vi "NI_low_level_daq_analog_waveform_generator.vi"() -> ()   [LabVIEW 2025]
uses:
  <vilib>/DAQmx/write.llb/DAQmx Write (Analog 2D DBL NChan NSamp).vi
  <vilib>/DAQmx/create/channels.llb/DAQmx Create Channel (AO-Voltage-Basic).vi
  <vilib>/DAQmx/configure/timing.llb/DAQmx Timing (Sample Clock).vi
  <vilib>/DAQmx/miscellaneous.llb/DAQmx Fill In Error Info.vi
  <vilib>/measure/NI_MABase.lvlib
panel:
  in  "Number of Points":dbl=1000.0 format="%#_13g"
  in  "Sampling frequency":dbl=5000.0 format="%#_13g"
  in  "Together ON/OFF":bool
  out "Boolean":bool
  out "Boolean":bool
  in  "Output to DAQ":bool
  out "DAQ Output Voltage":waveform(dbl)[](graph)
  in  "Voltage Amplitude":i32=1 min=0 max=10 step=1
  in  "Frequency (Hz)":i32=10
  in  "Phase (degrees)":i32
  in  "Waveform":string(combo)="sine"
  in  "Phase (degrees)":i32
  in  "Waveform":string(combo)="sine"
  in  "Frequency (Hz)":i32=10
  in  "Voltage Amplitude":i32=1 min=0 max=10 step=1
  in  "stop":bool
  # "Waveform Generator (open-loop)"
  # "X-AXIS"
  # "Y-AXIS"
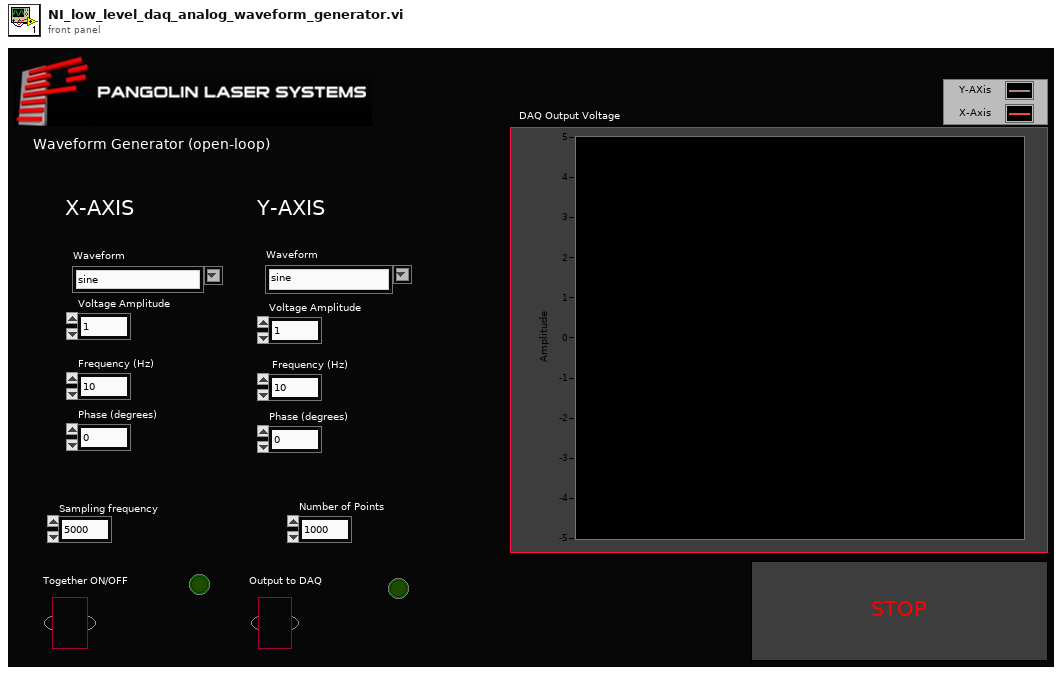
[diagram p1: front panel]
types:
  T1 = cluster{"Sampling frequency":dbl, "Number of Points":dbl}
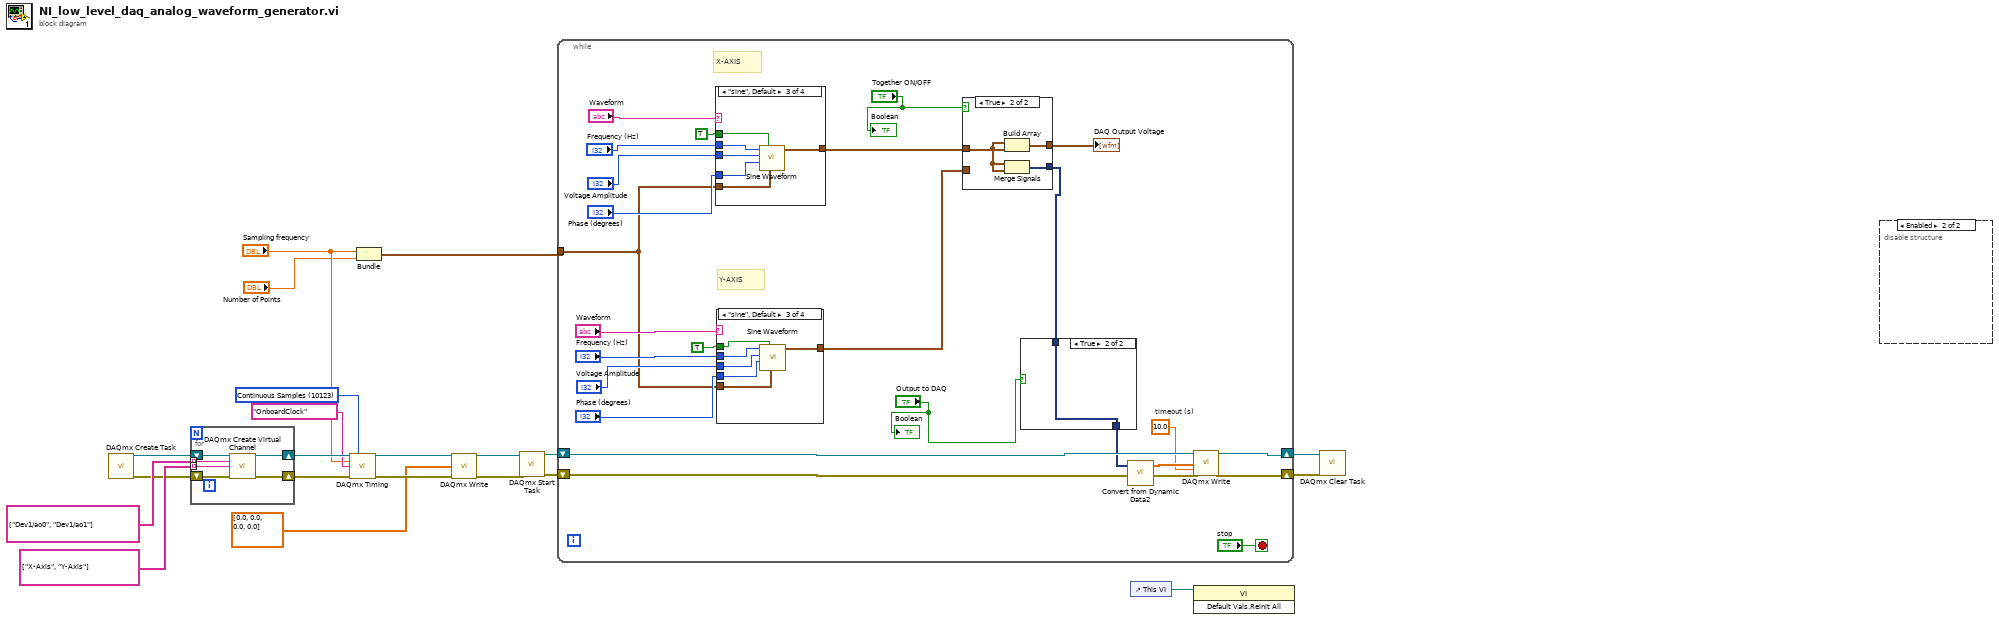
[diagram p0: block diagram]
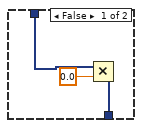
[diagram p2: hidden frame]
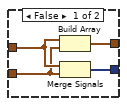
[diagram p3: hidden frame]
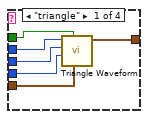
[diagram p4: hidden frame]
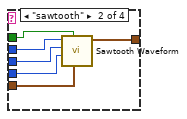
[diagram p5: hidden frame]
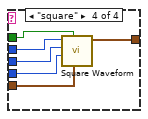
[diagram p6: hidden frame]
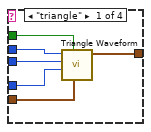
[diagram p7: hidden frame]
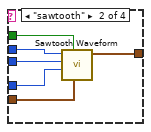
[diagram p8: hidden frame]
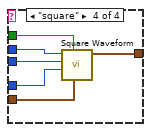
[diagram p9: hidden frame]
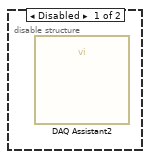
[diagram p10: hidden frame]
diagram:
  w14 = 10123 items=["Finite Samples"=10178, "Continuous Samples"=10123, "Hardware Timed Single Point"=12522] ("sample mode")
  n1 = call <vilib>:"DAQmx Create Task.vi"() -> ("task out"=w17:refnum<k21>, "error out"=w18:errorcluster)  [unwired: 14 in]
  n2 = for {
    tunnel: tag[] ["Dev1/ao0", "Dev1/ao1"] ("physical channels") -> [w27] mode=indexing
    tunnel: string[] ["X-Axis", "Y-Axis"] ("name to assign") -> [w26] mode=indexing
    shift-right: [w22] -> w15
    shift-left: w18 -> [w25]
    shift-right: [w23] -> w16
    shift-left: w17 -> [w24]
    n3 = call-poly <vilib>:"DAQmx Create Virtual Channel.vi"("task in"=w24, "physical channels"=w27, "name to assign"=w26, "error in"=w25) -> ("task out"=w23:refnum<k21>, "error out"=w22:errorcluster)  [unwired: 10 in]
  }
  n4 = call-poly <vilib>:"DAQmx Timing.vi"("task/channels in"=w16, "sample mode"=w14, "rate"="Sampling frequency", "source"=tag "OnboardClock", "error in"=w15) -> ("task out"=w11:refnum<k21>, "error out"=w10:errorcluster)  [unwired: 9 in]
  n5 = Bundle("Sampling frequency"="Sampling frequency", "Number of Points"="Number of Points") -> (w1:T1)  [unwired: 1 in]
  n6 = call-poly <vilib>:"DAQmx Write.vi"("task/channels in"=w11, "data"=dbl[][] [[0.0, 0.0], [0.0, 0.0]], "error in"=w10) -> ("task out"=w13:refnum<k21>, "error out"=w12:errorcluster)  [unwired: 10 in, 1 out]
  n7 = call <vilib>:"DAQmx Start Task.vi"("task/channels in"=w13, "error in"=w12) -> ("task out"=w8:refnum<k21>, "error out"=w6:errorcluster)  [unwired: 12 in]
  n8 = while {
    tunnel: w1 -> [w40]
    shift-right: [w50] -> w5
    shift-left: w8 -> [w52]
    shift-right: [w49] -> w4
    shift-left: w6 -> [w51]
    stop <- "stop" stop-if-true
    w30 = 10.0  # timeout (s)
    # "Y-AXIS"
    # "X-AXIS"
    n9 = case shown="\"sine\", Default" "Waveform" {
      tunnel: "Voltage Amplitude" -> [w92 w98 w104 w111]
      tunnel: "Frequency (Hz)" -> [w93 w99 w105 w110]
      tunnel: w40 -> [w89 w95 w102 w109]
      tunnel: [w90 w94 w101 w108] -> w38
      tunnel: "Phase (degrees)" -> [w91 w97 w103 w107]
      tunnel: TRUE ("reset signal") -> [w88 w96 w100 w106]
      frame "triangle" {
        n10 = call <vilib>:"Triangle Waveform.vi"("sampling info"=w89, "reset signal"=w88, "phase"=w91, "amplitude"=w92, "frequency"=w93) -> ("signal out"=w90:waveform(dbl))  [unwired: 5 in, 1 out]
      }
      frame "sawtooth" {
        n11 = call <vilib>:"Sawtooth Waveform.vi"("sampling info"=w95, "reset signal"=w96, "phase"=w97, "amplitude"=w98, "frequency"=w99) -> ("signal out"=w94:waveform(dbl))  [unwired: 5 in, 1 out]
      }
      frame "sine", Default {
        n12 = call <vilib>:"Sine Waveform.vi"("sampling info"=w102, "reset signal"=w100, "phase"=w103, "amplitude"=w104, "frequency"=w105) -> ("signal out"=w101:waveform(dbl))  [unwired: 5 in, 1 out]
      }
      frame "square" {
        n13 = call <vilib>:"Square Waveform.vi"("sampling info"=w109, "reset signal"=w106, "phase"=w107, "amplitude"=w111, "frequency"=w110) -> ("signal out"=w108:waveform(dbl))  [unwired: 5 in, 1 out]
      }
    }
    n14 = case shown="\"sine\", Default" "Waveform" {
      tunnel: "Voltage Amplitude" -> [w67 w74 w79 w87]
      tunnel: "Frequency (Hz)" -> [w68 w75 w80 w86]
      tunnel: w40 -> [w64 w71 w77 w85]
      tunnel: [w65 w70 w76 w84] -> w37
      tunnel: TRUE ("reset signal") -> [w69 w72 w81 w83]
      tunnel: "Phase (degrees)" -> [w66 w73 w78 w82]
      frame "triangle" {
        n15 = call <vilib>:"Triangle Waveform.vi"("sampling info"=w64, "reset signal"=w69, "phase"=w66, "amplitude"=w67, "frequency"=w68) -> ("signal out"=w65:waveform(dbl))  [unwired: 5 in, 1 out]
      }
      frame "sawtooth" {
        n16 = call <vilib>:"Sawtooth Waveform.vi"("sampling info"=w71, "reset signal"=w72, "phase"=w73, "amplitude"=w74, "frequency"=w75) -> ("signal out"=w70:waveform(dbl))  [unwired: 5 in, 1 out]
      }
      frame "sine", Default {
        n17 = call <vilib>:"Sine Waveform.vi"("sampling info"=w77, "reset signal"=w81, "phase"=w78, "amplitude"=w79, "frequency"=w80) -> ("signal out"=w76:waveform(dbl))  [unwired: 5 in, 1 out]
      }
      frame "square" {
        n18 = call <vilib>:"Square Waveform.vi"("sampling info"=w85, "reset signal"=w83, "phase"=w82, "amplitude"=w87, "frequency"=w86) -> ("signal out"=w84:waveform(dbl))  [unwired: 5 in, 1 out]
      }
    }
    n19 = case shown="True" "Together ON/OFF" {
      tunnel: w38 -> [w60 w61]
      tunnel: w37 -> [w59 _]
      tunnel: [w58 w63] -> w32
      tunnel: [w57 w62] -> w36
      frame False {
        n20 = Build Array(w60, w59) -> (w57:waveform(dbl)[])
        n21 = Merge Signals(w60, w59) -> (w58:dynamicdata)
      }
      frame True {
        n22 = Build Array(w61, w61) -> (w62:waveform(dbl)[])
        n23 = Merge Signals(w61, w61) -> (w63:dynamicdata)
      }
    }
    "DAQ Output Voltage" <- w36
    n24 = case shown="True" "Output to DAQ" {
      tunnel: w32 -> [w55 w56]
      tunnel: [w53 w56] -> w29
      frame False {
        n25 = Multiply(x=w55, y=0.0) -> (x*y=w53:dynamicdata)
      }
      frame True {
      }
    }
    n26 = call "Convert from Dynamic Data2"("Dynamic Data Type"=w29) -> ("Array"=w31:dbl[][])  [unwired: 3 in]
    n27 = call-poly <vilib>:"DAQmx Write.vi"("task/channels in"=w52, "data"=w31, "timeout"=w30, "error in"=w51) -> ("task out"=w50:refnum<k21>, "error out"=w49:errorcluster)  [unwired: 9 in, 1 out]
    "Boolean" <- "Output to DAQ"
    "Boolean" <- "Together ON/OFF"
  }
  n28 = control-ref of="This VI"() -> (w21:refnum<vi>)
  n29 = invoke class="VI" method="Default Vals.Reinit All"(reference=w21) -> ()  [unwired: 2 in, 3 out]
  n30 = call <vilib>:"DAQmx Clear Task.vi"("task in"=w5, "error in"=w4) -> ()  [unwired: 13 in, 1 out]
  n31 = disable-structure shown="Enabled" {
    frame Disabled {
      n32 = call "DAQ Assistant2"() -> ()  [unwired: 17 in, 3 out]
    }
    frame Enabled {
    }
  }
